vi "Enable Disable Progress Bar on helper loop.vi"(10 "Enable":bool, 11 "Progress bar":refnum<vi>) -> ()   [LabVIEW 2019, in "Panther Dashboard.lvlib"]
uses:
  Panther Dashboard.lvlib
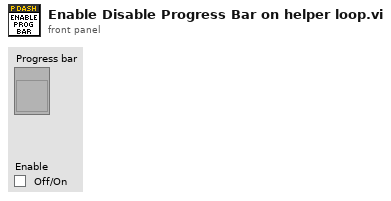
[diagram p1: front panel]
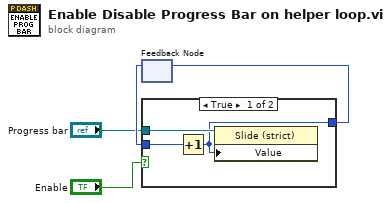
[diagram p0: block diagram]
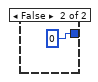
[diagram p2: hidden frame]
diagram:
  n1 = feedback #1() -> (w2:u8)  [unwired: 1 in]
  n2 = case shown="True" "Enable" {
    tunnel: "Progress bar" -> [w7 _]
    tunnel: [w6 u8 0 ("Value")] -> w3
    tunnel: w2 -> [w5 _]
    frame True {
      n3 = Increment(x=w5) -> (x+1=w6:u8)
      n4 = property class="Slide (strict)"(reference=w7, "Value"=w6) -> ()  [unwired: 1 in, 2 out]
    }
    frame False {
    }
  }
  n5 = feedback-in #1(w3) -> ()
